vi "MAIN_RX.vi"() -> ()   [LabVIEW 2017]
panel:
  out "Progress":u32(slide) scale=0.0..100.0
  in  "simbol per cycle":i32=120
  out "image out":T1(plugin-control)
  out "received symbols":i32[](array[numeric])
  in  "level":dbl=0.01 format="%#_13g"
  out "size(s)":i32=375000
  in  "heigth":i32=125
  in  "width":i32=125
  in  "color":bool=TRUE
  in  "IQ Rate [S/sec]":dbl=2000000.0 format="%#_6p"
  in  "pulse duration[sample]":i32=5
  in  "M":i8=16
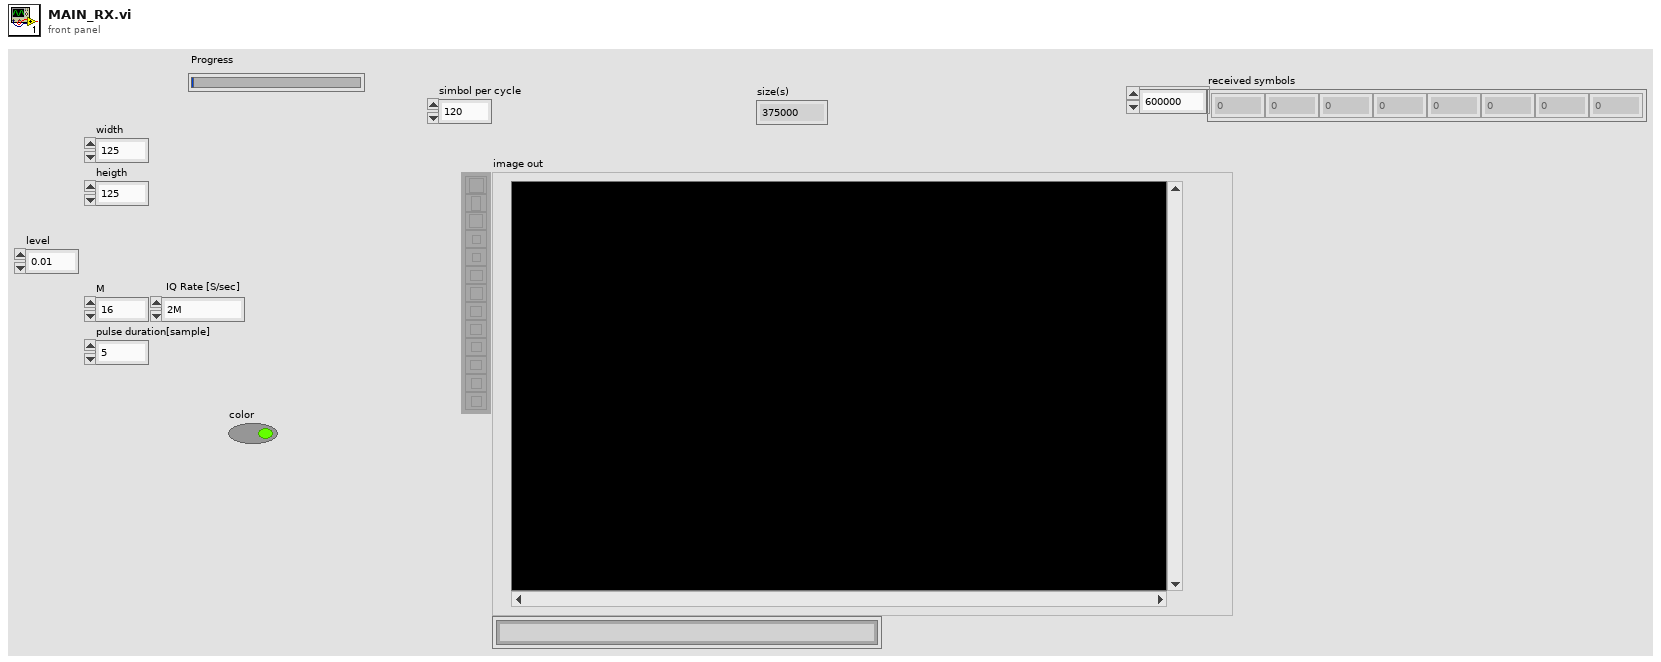
[diagram p1: front panel]
types:
  T1 = typedef "IMAQ Image.ctl" = refnum<image>
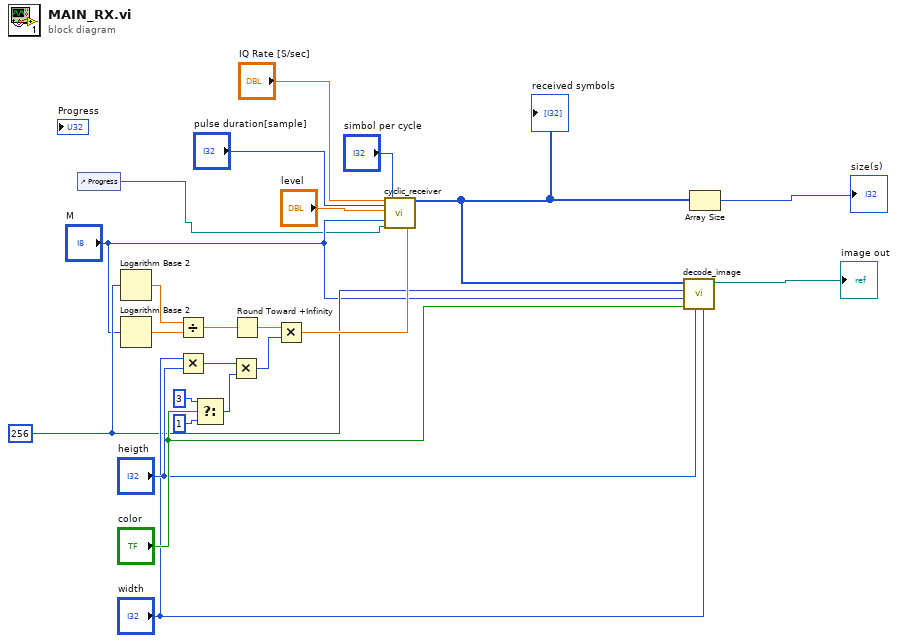
[diagram p0: block diagram]
diagram:
  w8 = i16 256 ("max")
  n1 = control-ref of="Progress"() -> (w1:refnum<vi>)
  n2 = Logarithm Base 2(1:w8) -> (0:w6:dbl)
  n3 = Logarithm Base 2(1:"M") -> (0:w5:dbl)
  n4 = Divide(x=w6, y=w5) -> (x/y=w4:dbl)
  n5 = Multiply(x="width", y="heigth") -> (x*y=w19:i32)
  n6 = Select(t=i8 3 ("y"), s="color", f=i8 1) -> (s? t:f=w20:i8)
  n7 = Multiply(x=w19, y=w20) -> (x*y=w11:i32)
  n8 = Round Toward +Infinity(x=w4) -> (ceil(x): smallest int >= x=w3:dbl)
  n9 = Multiply(x=w3, y=w11) -> (x*y=w10:dbl)
  n10 = call "cyclic_receiver.vi"("IQ Rate [S/sec]"="IQ Rate [S/sec]", "pulse duration[sample]"="pulse duration[sample]", "level"="level", "M"="M", "reference"=w1, "Symbol per cycle"="simbol per cycle", "simboli da ricevere"=w10) -> ("received symbols"=w13:i8[])  [unwired: 10 in, 2 out]
  "received symbols" <- w13
  n11 = call "decode_image.vi"("width"="width", "heigth"="heigth", "Color"="color", "M"="M", "max"=w8, "Array"=w13) -> ("image out"=→"image out":T1)  [unwired: 4 in, 1 out]
  n12 = Array Size(array=w13) -> (size(s)=→"size(s)":i32)
